vi "Stop.vi"(0 "reference in":refnum<class "MLA.lvclass">, 5 "error in (no error)":errorcluster) -> (14 "reference out":refnum<class "MLA.lvclass">, 19 "error out":errorcluster)   [LabVIEW 2023, in "MLA.lvclass"]
uses:
  MLA.lvclass
  MLA Stop Mode.ctl
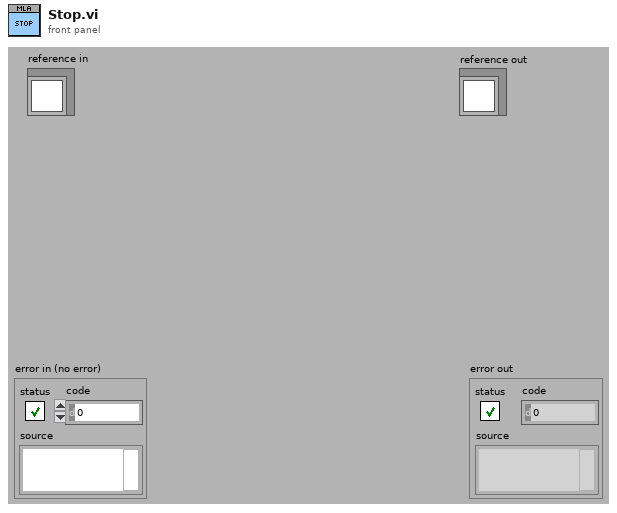
[diagram p1: front panel]
types:
  T1 = typedef "MLA Stop Mode.ctl" = enum16{"Read", "Set", "Reset"}
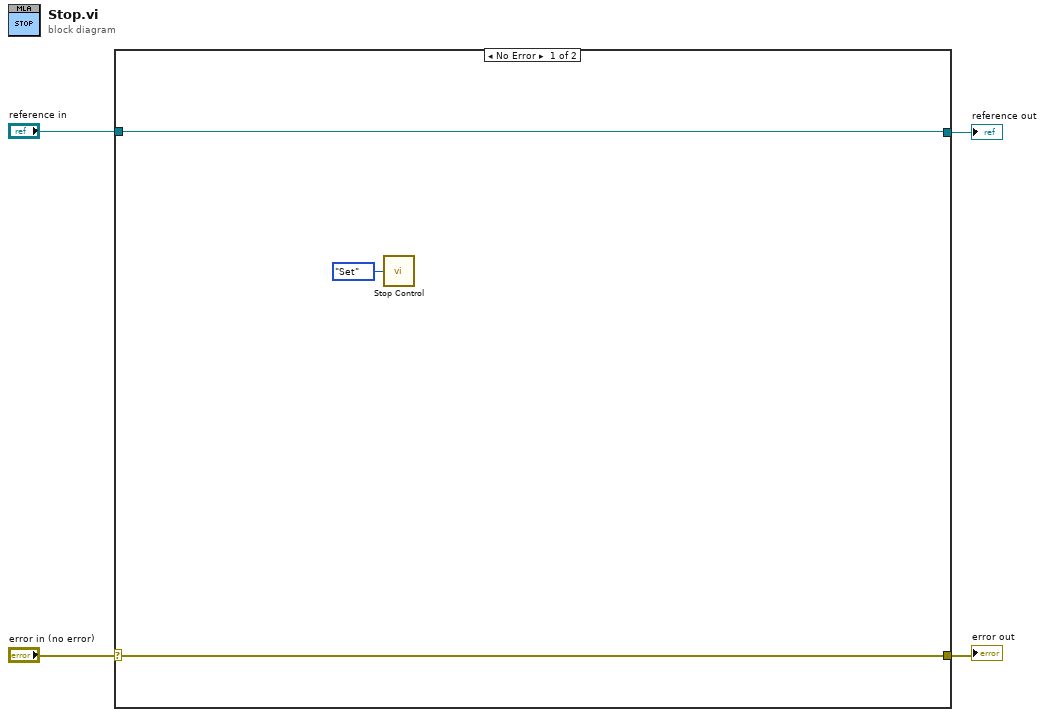
[diagram p0: block diagram]
diagram:
  n1 = case shown="No Error" "error in (no error)" {
    selector: "error in (no error)" -> [w5 w9]
    tunnel: [w5 w9] -> w3
    tunnel: [w7 w8] -> w1
    tunnel: "reference in" -> [w7 w8]
    frame No Error {
      n2 = call "Stop Control.vi"("Mode (Read)"=MLA_Stop_Mode."Set") -> ()  [unwired: 1 out]
    }
    frame Error {
    }
  }
  "error out" <- w3
  "reference out" <- w1
